vi "remove tag from default data table.vi"(9 "index":i32, 10 "data type":T1, 11 "data dictionary in":refnum<class "data dictionary.lvclass">) -> (3 "data dictionary out":refnum<class "data dictionary.lvclass">)   [LabVIEW 2013, in "tag bus.lvlib" / "data dictionary.lvclass"]
doc: "Removes a data element from the default data table."
uses:
  data dictionary.lvclass
  tag/Data Type.ctl
  data dictionary.lvclass/data dictionary.ctl
  table/data table.lvlib
  tag/tag descriptor.lvclass
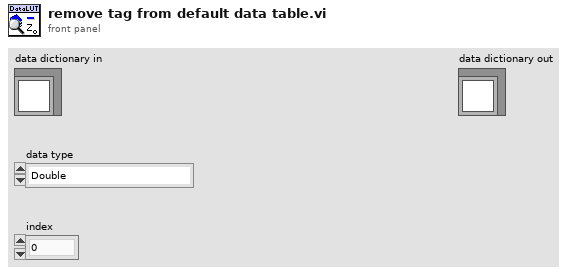
[diagram p1: front panel]
types:
  T1 = typedef "tag bus.lvlib/tag descriptor.lvclass/Data Type.ctl" = enum16{"Double", "Single", "I64", "I32", "I16", "I8", "U64", "U32", "U16", "U8", "Boolean", "String", "Array of Double", "Array of Single", "Array of I64", "Array of I32", "Array of I16", "Array of I8", "Array of U64", "Array of U32", "Array of U16", "Array of U8", "Array of Boolean", "Array of String"}
  T2 = typedef "tag bus.lvlib/data table.lvlib/data table.ctl" = cluster{"Double":dbl[], "Single":sgl[], "I64":i64[], "I32":i32[], "I16":i16[], "I8":i8[], "U64":u64[], "U32":u32[], "U16":u16[], "U8":u8[], "Boolean":bool[], "String":string[], "Array of Double":cluster{"DBL Array":dbl[]}[], "Array of Single":cluster{"SGL Array":sgl[]}[], "Array of I64":cluster{"I64 Array":i64[]}[], "Array of I32":cluster{"I32 Array":i32[]}[], "Array of I16":cluster{"I16 Array":i16[]}[], "Array of I8":cluster{"I8 Array":i8[]}[], "Array of U64":cluster{"U64 Array":u64[]}[], "Array of U32":cluster{"U32 Array":u32[]}[], "Array of U16":cluster{"U16 Array":u16[]}[], "Array of U8":cluster{"U8 Array":u8[]}[], "Array of Boolean":cluster{"Boolean Array":bool[]}[], "Array of String":cluster{"String Array":string[]}[]}
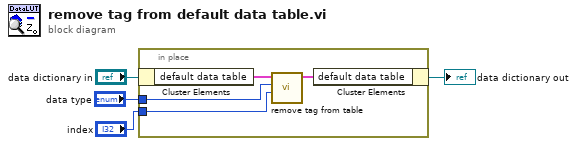
[diagram p0: block diagram]
diagram:
  n1 = in-place {
    in-place-border: "data type" -> [w7]
    in-place-border: "index" -> [w5]
    n2 = in-place-cluster #1("data dictionary in") -> ("default data table"=w8:T2)
    n3 = call "remove tag from table.vi"("index"=w5, "data type"=w7, "data table in"=w8) -> ("data table out"=w6:T2)  [unwired: 8 in]
    n4 = in-place-cluster #1("default data table"=w6) -> (→"data dictionary out":refnum<class "data dictionary.lvclass">)
  }
